vi "Autoaim.vi"(8 "Autoaim":bool, 10 "Target":T1 {"Orientation" format="%.2f"; "Dimensions"."Height" format="%.2f"; "Dimensions"."Width" format="%.2f"; "Center of Mass"."Y" format="%.2f"; "Center of Mass"."X" format="%.2f"; "Bounding Rect"."Bottom" format="%.2f"; "Bounding Rect"."Right" format="%.2f"; "Bounding Rect"."Top" format="%.2f"; "Bounding Rect"."Left" format="%.2f"; "Number of Holes" format="%.2f"; "Area" format="%.2f"}) -> (0 "Fire":bool, 1 "Motor Output":dbl, 3 "Rotation":dbl)   [LabVIEW 2013]
uses:
  Utils/Target Type.ctl
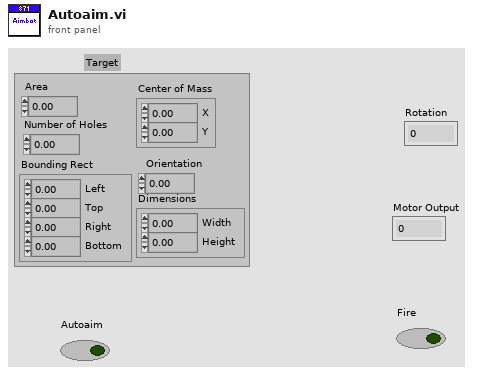
[diagram p1: front panel]
types:
  T1 = typedef "Target Type.ctl" = cluster{"Area":dbl, "Number of Holes":dbl, "Bounding Rect":cluster{"Left":dbl, "Top":dbl, "Right":dbl, "Bottom":dbl}, "Center of Mass":cluster{"X":dbl, "Y":dbl}, "Orientation":dbl, "Dimensions":cluster{"Width":dbl, "Height":dbl}}
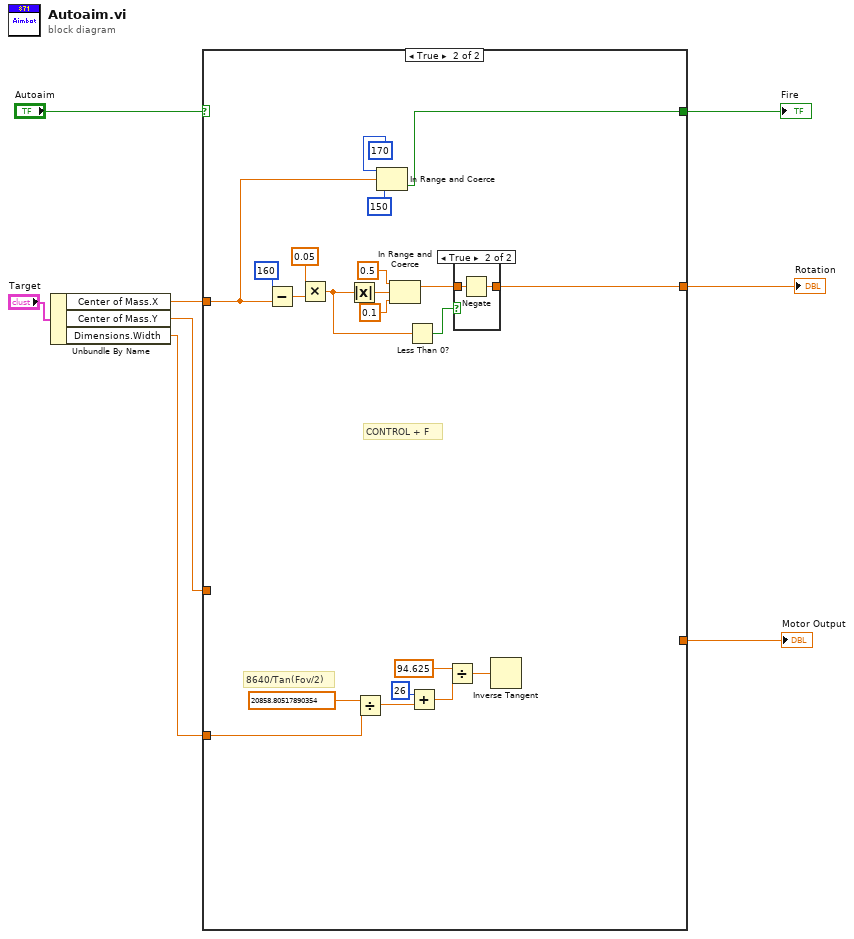
[diagram p0: block diagram]
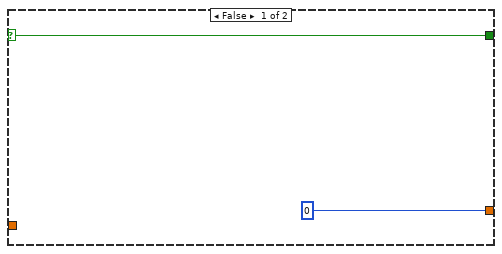
[diagram p2: hidden frame]
diagram:
  n1 = Unbundle By Name("Target") -> ("Center of Mass.X"=w6:dbl, "Center of Mass.Y"=w3:dbl, "Dimensions.Width"=w2:dbl)
  n2 = case shown="True" "Autoaim" {
    selector: "Autoaim" -> [w9 _]
    tunnel: w6 -> [_ w19]
    tunnel: [0 w22] -> w5
    tunnel: [w9 w18] -> w4
    tunnel: w3 -> [_ _]
    tunnel: w2 -> [_ w16]
    tunnel: [_ _] -> w1
    frame False {
    }
    frame True {
      # "CONTROL + F"
      # "8640/Tan(Fov/2)"
      n3 = Subtract(x=160, y=w19) -> (x-y=w29:dbl)
      n4 = Multiply(x=0.05, y=w29) -> (x*y=w23:dbl)
      n5 = Absolute Value(x=w23) -> (abs(x)=w26:dbl)
      n6 = Divide(x=20858.80517890354, y=w16) -> (x/y=w12:dbl)
      n7 = In Range and Coerce(upper limit=170, x=w19, lower limit=150) -> (In Range?=w18:bool)  [unwired: 1 out]
      n8 = In Range and Coerce(upper limit=0.5, x=w26, lower limit=0.1) -> (coerced(x)=w24:dbl)  [unwired: 1 out]
      n9 = Less Than 0?(x=w23) -> (x < 0?=w25:bool)
      n10 = Add(x=26, y=w12) -> (x+y=w11:dbl)
      n11 = Divide(x=94.625, y=w11) -> (x/y=w14:dbl)
      n12 = case shown="True" w25 {
        tunnel: w24 -> [w32 w34]
        tunnel: [w32 w33] -> w22
        frame False {
        }
        frame True {
          n13 = Negate(x=w34) -> (-x=w33:dbl)
        }
      }
      n14 = Inverse Tangent(1:w14) -> ()  [unwired: 1 out]
    }
  }
  "Fire" <- w4
  "Rotation" <- w5
  "Motor Output" <- w1
